vi "Main.vi"() -> ()   [LabVIEW 2014, in "CSV Analyzer.lvlib"]
uses:
  CSV Analyzer.lvlib
  <vilib>/SLL/SLL Table/SLL Table.lvclass
  <vilib>/Utility/error.llb/DialogType.ctl
  <vilib>/SLL/SLL Queued State Machine/Queue Driver/Create Queue.vi
  <vilib>/SLL/SLL Queued State Machine/Queue Driver/Enqueue an Item to Queue.vi
  <vilib>/SLL/SLL Queued State Machine/Queue Driver/Dequeue Queue.vi
  <vilib>/Utility/file.llb/Read From Spreadsheet File (string).vi
  <vilib>/SLL/SLL Queued State Machine/Queue Driver/Enqueue N Items.vi
  <vilib>/SLL/SLL Queued State Machine/Queue Driver/Flush Queue.vi
  <vilib>/SLL/SLL Queued State Machine/Queue Driver/Release Queue.vi
  <vilib>/SLL/SLL Queued State Machine/SLL QSM.lvlib
  <vilib>/SLL/SLL Spreadsheet/SLL Spreadsheet.lvlib
panel:
  in  "Delimiter":string(combo)=","
  in  "Use LabVIEW File Read?":bool
  in  "CSV File Path":path
  out "Total Columns":i32
  out "Total Rows":i32
  in  "Headers to List[]":string[](array[combo])
  in  "Filters":T1(array[cluster])
  out "Status":string
  in  "Analyze":bool
  out "Displayed Column Count":i32
  out "Displayed Row Count":i32
  in  "Mini Table":bool
  in  "2D Data Out[][]":i32(listbox)
  # "CSV Analyzer"
  # "Empty: Displays All Columns"
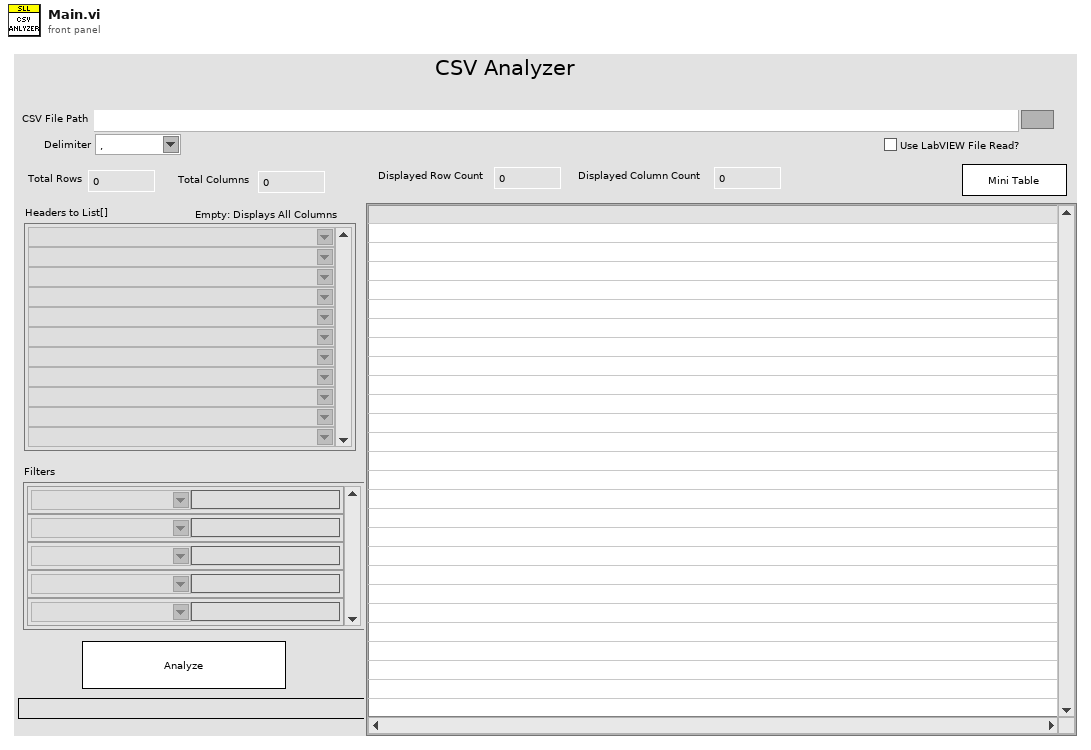
[diagram p1: front panel]
types:
  T1 = cluster{"Enable?":string, "Column Name":string}[]
  T2 = cluster{"Flags":cluster{"Source Code?":bool}, "SLL Table":refnum<class "SLL Table.lvclass">, "Headers[]":string[]}
  T3 = typedef "DialogType.ctl" = u16
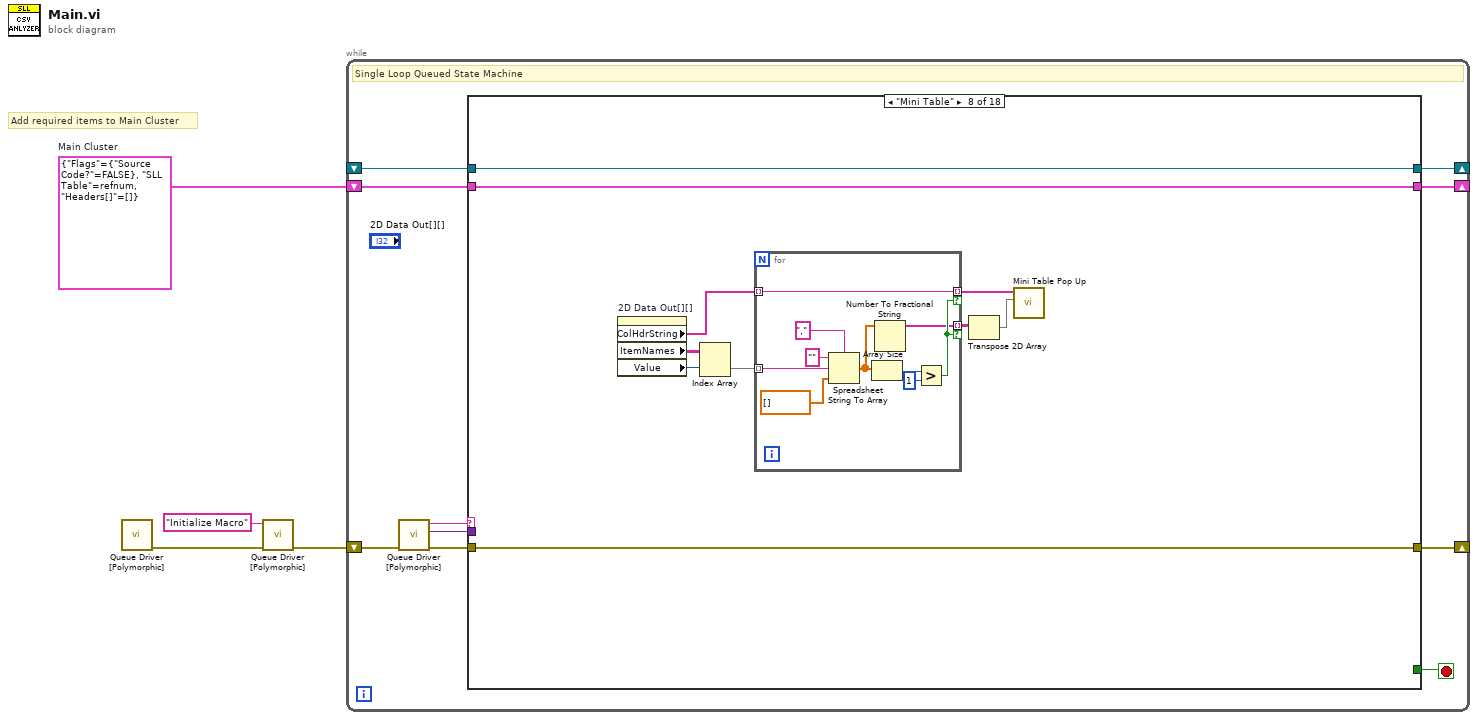
[diagram p0: block diagram]
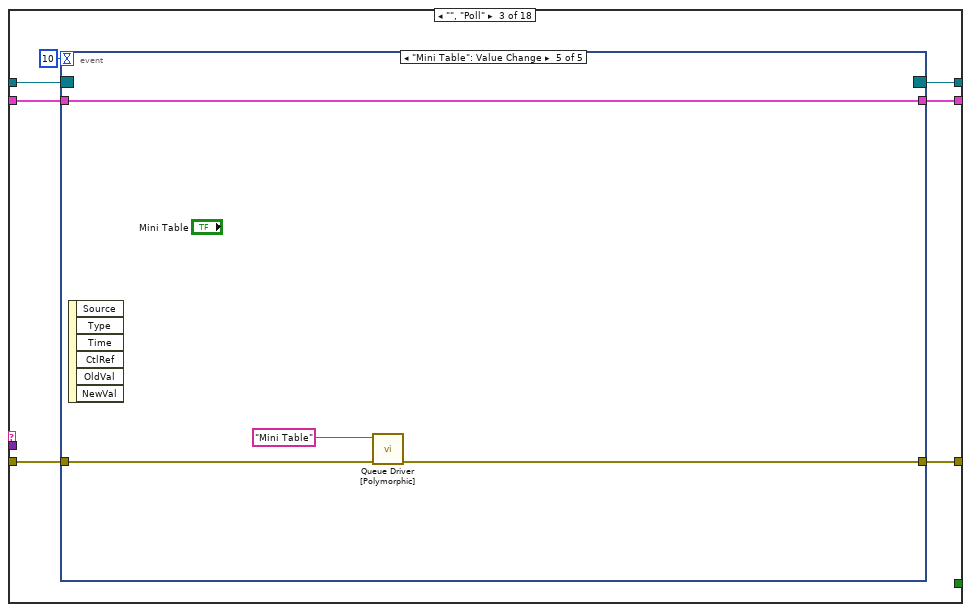
[diagram p4: hidden frame]
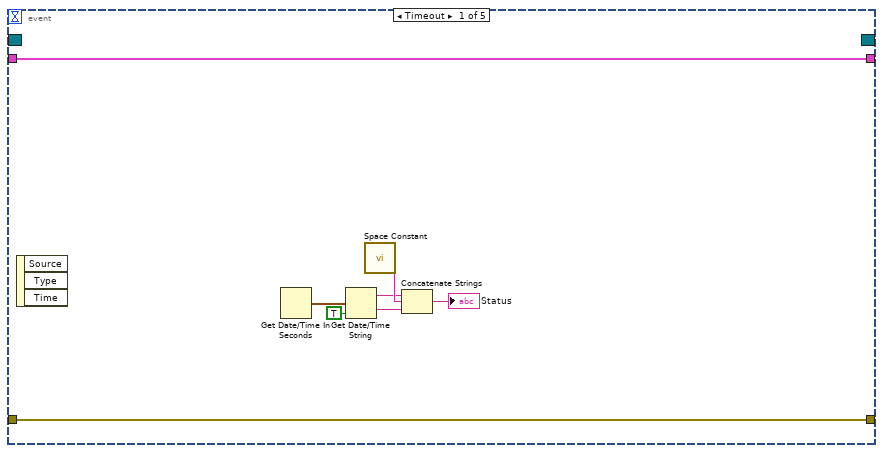
[diagram p5: hidden frame]
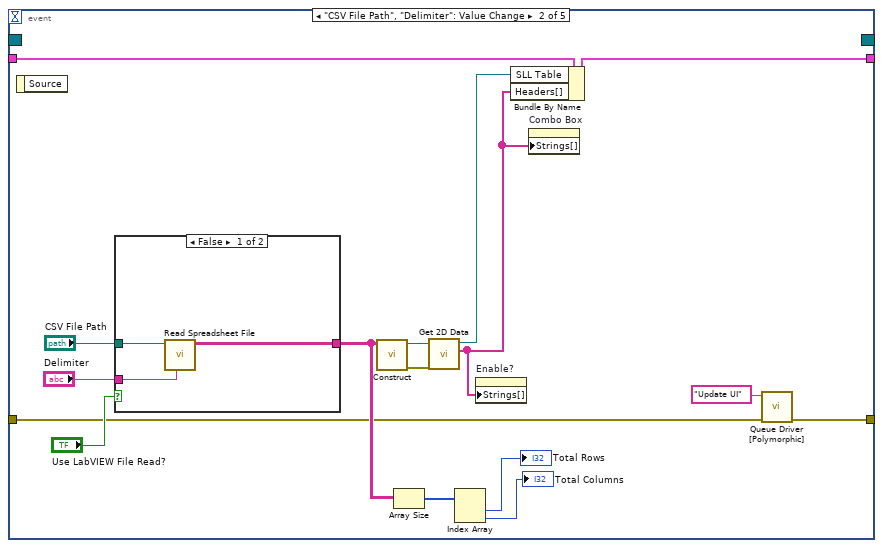
[diagram p6: hidden frame]
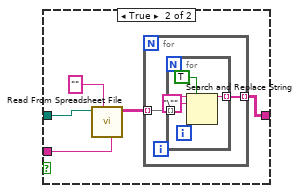
[diagram p7: hidden frame]
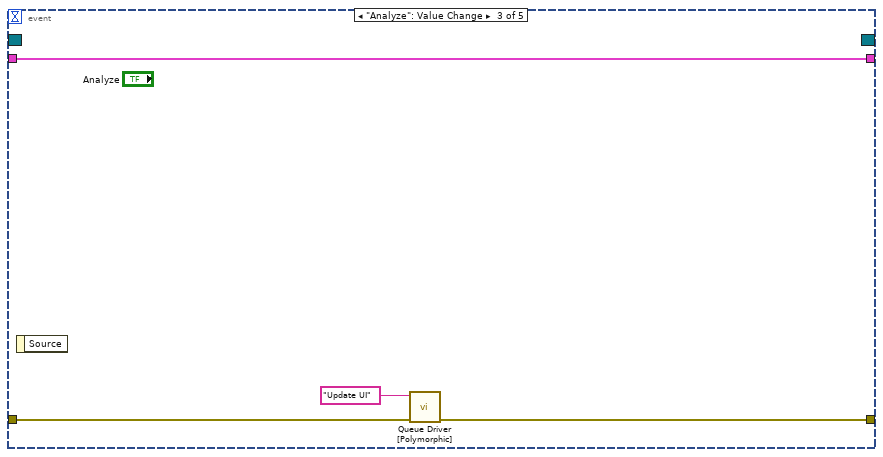
[diagram p8: hidden frame]
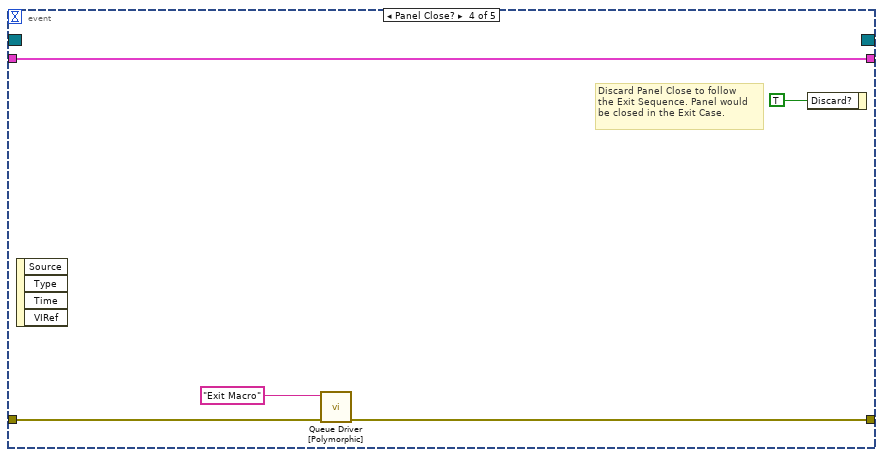
[diagram p9: hidden frame]
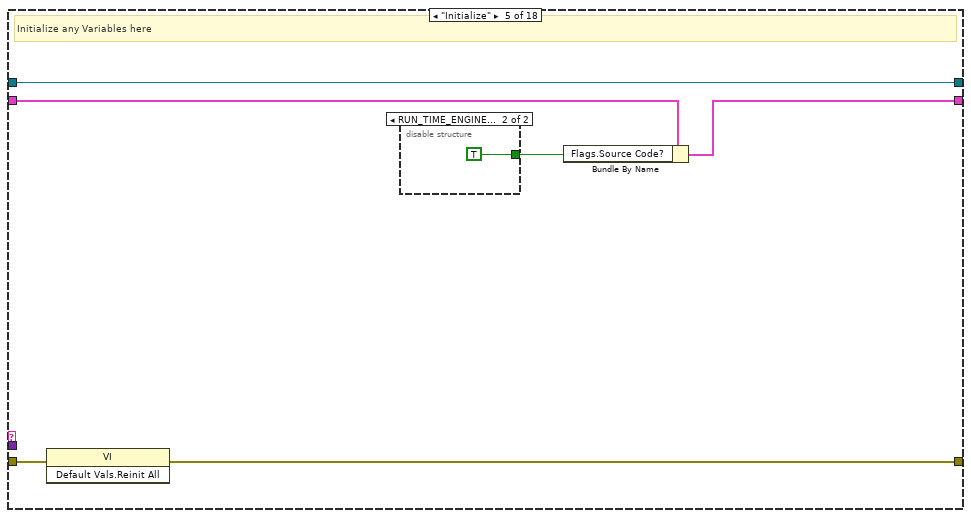
[diagram p11: hidden frame]
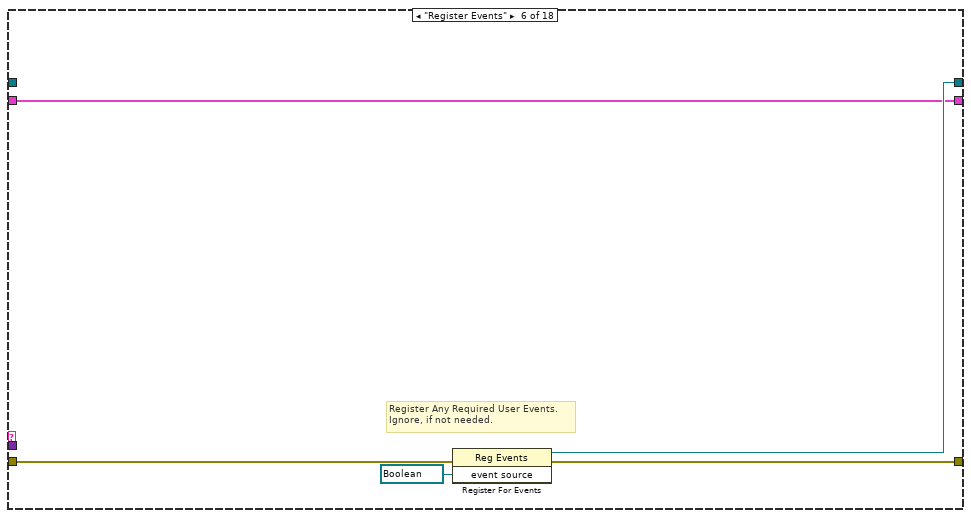
[diagram p13: hidden frame]
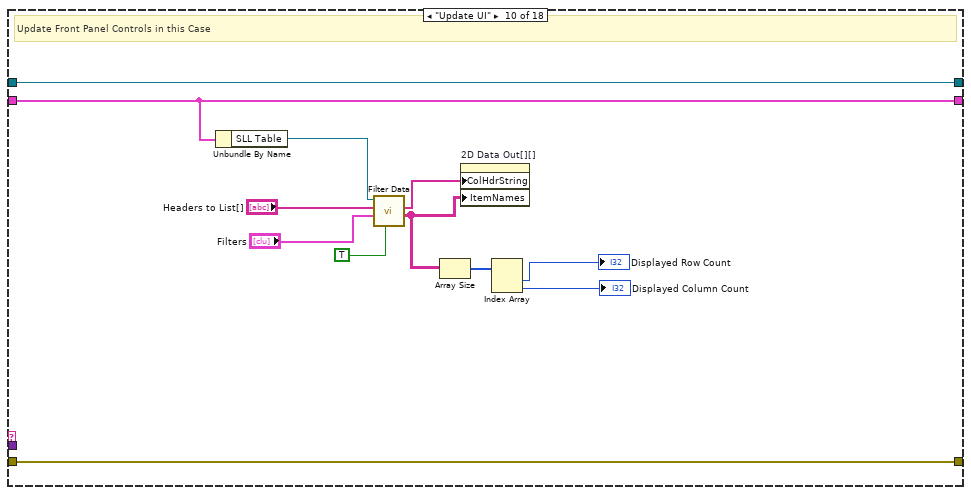
[diagram p16: hidden frame]
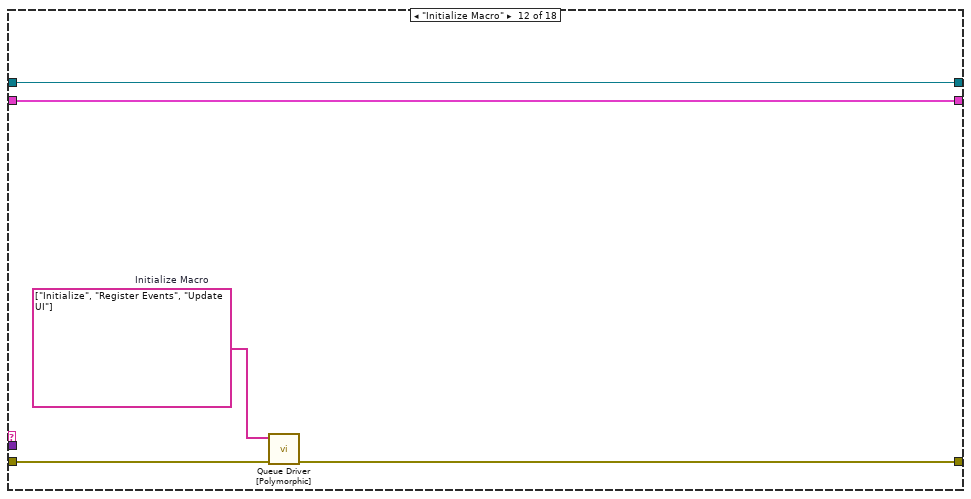
[diagram p18: hidden frame]
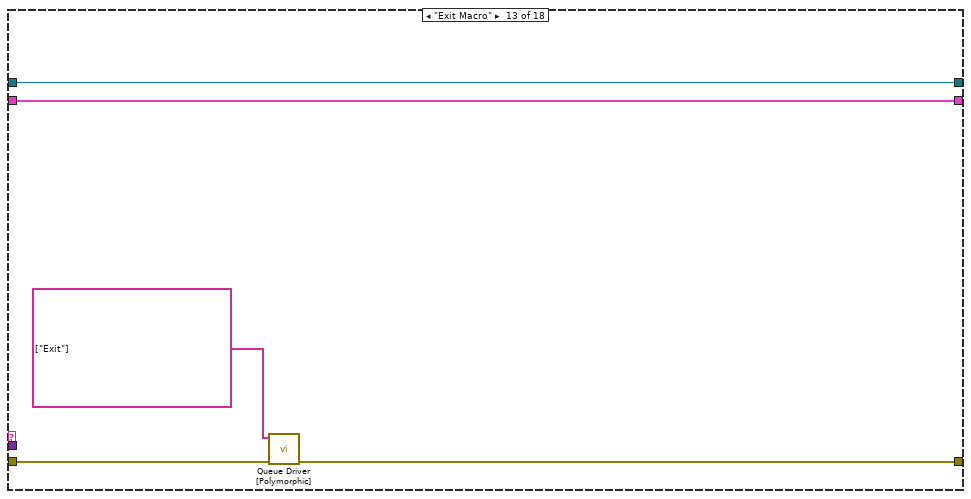
[diagram p19: hidden frame]
diagram:
  w3 = T2 {"Flags"={"Source Code?"=FALSE}, "SLL Table"=refnum, "Headers[]"=[]}  # Main Cluster
  # "Add required items to Main Cluster"
  n1 = call-poly <vilib>:"Queue Driver [Polymorphic].vi"() -> ("Error Out"=w2:errorcluster)  [unwired: 11 in]
  n2 = call-poly <vilib>:"Queue Driver [Polymorphic].vi"("Error In"=w2, "Item to Add"="Initialize Macro") -> ("Error Out"=w1:errorcluster)  [unwired: 9 in]
  n3 = while "SLL Queued State Machine" {
    shift-right: [w12] -> _
    shift-left: w1 -> [w14]
    shift-right: [w9] -> _
    shift-left: _ -> [w8]
    shift-right: [w7] -> _
    shift-left: w3 -> [w6]
    stop <- w11 stop-if-true
    # "Single Loop Queued State Machine"
    n4 = call-poly <vilib>:"Queue Driver [Polymorphic].vi"("Error In"=w14) -> ("Error Out"=w13:errorcluster, "Data"=w5:variant, "Dequeue"=w10:string)  [unwired: 8 in]
    n5 = case "QSM Case Structure" shown="\"Mini Table\"" w10 {
      selector: w10 -> [_ _ _ _ _ _ _ _ _ _ _ _ _ _ w151 _ _ _]
      tunnel: w13 -> [w17 w20 w25 w81 w82 w93 w96 w106 w119 w131 w134 w137 w142 w147 w150 w163 w166 w179]
      tunnel: [w17 w20 w26 w81 w83 w92 w96 w106 w119 w131 w134 w136 w141 w147 w154 w161 w166 w175] -> w12
      tunnel: [_ _ _ _ _ _ _ _ _ _ _ _ _ _ _ _ _ TRUE] -> w11
      tunnel: [w16 w19 w24 w80 w87 w91 w95 w105 w118 w130 w133 w139 w144 w146 w157 w160 w165 w178] -> w9
      tunnel: w8 -> [w16 w19 w23 w80 w87 _ w95 w105 w118 w130 w133 w139 w144 w146 w157 w160 w165 w178]
      tunnel: [w15 w18 w21 w79 w84 w90 w94 w104 w117 w120 w132 w138 w143 w145 w156 w159 w164 w177] -> w7
      tunnel: w6 -> [w15 w18 w22 w79 w85 w90 w94 w104 w117 w120 w132 w138 w143 w145 w156 w159 w164 w177]
      tunnel: w5 -> [_ _ _ _ _ _ _ _ _ _ _ _ _ _ _ _ _ _]
      frame "/--------------- Read Me -----------------/" {
        # "General Purpose Queue Based State Machine for Any Use Case (main application, module, pop up message etc)\n\nAdvantages:\n1. No Need to Pass Queue References between Queue Driver VIs.\n2. This template can be safely used in multiple parallel running modules without any issues.\n3. This template can also be safely used even in cases where the VI is configured to be a Clone, where multiple \ninstances of the VI could be executing concurrently.\n\nHow to Use:\n1. Add necessary items to the Main Cluster.\n2. Use the Polymorphic Queue Driver for doing any queue operations. There is no need to pass the queue driver\nreference, as the Queue Driver automatically infers the reference based on the VI instance from which it is called.\n3. Add any required user events in the \"Register Events\" case. Ignore if not needed.\n4. Use \"Sequences\" section for defining any list of state calls, which could be used in multiple places. \nEg: Initialize Sequence, might be needed if we need to any reinitialization."
      }
      frame "/------------------ Poll -------------------/" {
      }
      frame "", "Poll" {
        n6 = event shown="[4] \"Mini Table\": Value Change" {
          selector: w23 -> [_ _ _ _ _]
          dyn-events: [_ _ _ _ _] -> w24
          timeout: 10 -> [_ _ _ _ _]
          tunnel: [w35 w36 w67 w73 w77] -> w26
          tunnel: w25 -> [w35 w37 w66 w74 w78]
          tunnel: w22 -> [w34 w47 w69 w72 w76]
          tunnel: [w34 w49 w69 w72 w76] -> w21
          event Timeout {
            n7 = event-data() -> ()  [unwired: 1 in, 3 out]
            n8 = Get Date/Time In Seconds() -> (seconds since 1Jan1904=w33:timestamp)
            n9 = Get Date/Time String(seconds (now)=w33, want seconds? (F)=TRUE) -> (date string=w29:string, time string=w28:string)  [unwired: 1 in]
            n10 = call <vilib>:"Space Constant.vi"() -> ("String"=w30:string)
            n11 = Concatenate Strings(w29, w30, w28) -> (→"Status":string)
          }
          event "CSV File Path", "Delimiter": Value Change {
            n12 = event-data() -> ()  [unwired: 1 in, 1 out]
            n13 = case shown="False" "Use LabVIEW File Read?" {
              tunnel: [w54 w56] -> w45
              tunnel: "CSV File Path" -> [w53 w59]
              tunnel: "Delimiter" -> [w52 w55]
              frame False {
                n14 = call <vilib>:"Read Spreadsheet File.vi"("Delimiter (tab)"=w52, "File Path"=w53) -> ("2D Array"=w54:string[][])  [unwired: 8 in, 1 out]
              }
              frame True {
                n15 = call-poly <vilib>:"Read From Spreadsheet File.vi"("delimiter (\\t)"=w55, "format (%s)"="", "file path (dialog if empty)"=w59) -> ("all rows"=w57:string[][])  [unwired: 4 in, 4 out]
                n16 = for {
                  tunnel: w57 -> [w61] mode=indexing
                  tunnel: [w60] -> w56 mode=indexing
                  n17 = for {
                    tunnel: w61 -> [w65] mode=indexing
                    tunnel: [w63] -> w60 mode=indexing
                    n18 = Search and Replace String(replace all?=TRUE ("replace all? (F)"), input string=w65, search string="\"") -> (result string=w63:string)  [unwired: 5 in, 3 out]
                  }
                }
              }
            }
            n19 = call <vilib>:"Construct.vi"("2D String with Headers"=w45) -> ("error out"=w51:errorcluster, "SLL Spreadsheet"=w50:refnum<class "SLL Table.lvclass">)  [unwired: 9 in]
            n20 = Array Size(array=w45) -> (size(s)=w44:i32[])
            n21 = call <vilib>:"Get 2D Data.vi"("error in (no error)"=w51, "SLL Spreadsheet in"=w50) -> ("Headers Out[]"=w39:string[], "SLL Spreadsheet out"=w48:refnum<class "SLL Table.lvclass">)  [unwired: 6 in, 2 out]
            n22 = Index Array(array=w44) -> (element #1=→"Total Rows":i32, element #2=→"Total Columns":i32)  [unwired: 2 in]
            n23 = property on="Enable?" class="CmbBox"("Strings[]"=w39) -> ()  [unwired: 2 in, 2 out]
            n24 = Bundle By Name(cluster=w47, "SLL Table"=w48, "Headers[]"=w39) -> (w49:T2)
            n25 = property on="Combo Box" class="CmbBox"("Strings[]"=w39) -> ()  [unwired: 2 in, 2 out]
            n26 = call-poly <vilib>:"Queue Driver [Polymorphic].vi"("Error In"=w37, "Item to Add"="Update UI" ("Enqueue")) -> ("Error Out"=w36:errorcluster)  [unwired: 9 in]
          }
          event "Analyze": Value Change {
            n27 = event-data() -> ()  [unwired: 1 in, 1 out]
            n28 = call-poly <vilib>:"Queue Driver [Polymorphic].vi"("Error In"=w66, "Item to Add"="Update UI" ("Enqueue")) -> ("Error Out"=w67:errorcluster)  [unwired: 9 in]
          }
          event Panel Close? {
            # "Discard Panel Close to follow\nthe Exit Sequence. Panel would\nbe closed in the Exit Case."
            n29 = event-data() -> ()  [unwired: 1 in, 4 out]
            n30 = call-poly <vilib>:"Queue Driver [Polymorphic].vi"("Error In"=w74, "Item to Add"="Exit Macro" ("Enqueue")) -> ("Error Out"=w73:errorcluster)  [unwired: 9 in]
            n31 = event-data("Discard?"=TRUE) -> ()  [unwired: 1 in, 1 out]
          }
          event "Mini Table": Value Change {
            n32 = event-data() -> ()  [unwired: 1 in, 6 out]
            n33 = call-poly <vilib>:"Queue Driver [Polymorphic].vi"("Error In"=w78, "Item to Add"="Mini Table" ("Enqueue")) -> ("Error Out"=w77:errorcluster)  [unwired: 9 in]
          }
        }
      }
      frame "/--------------- Initialize -----------------/" {
      }
      frame "Initialize" {
        # "Initialize any Variables here"
        n34 = invoke class="VI" method="Default Vals.Reinit All"(error in=w82) -> (error out=w83:errorcluster)  [unwired: 2 in, 2 out]
        n35 = disable-structure shown="RUN_TIME_ENGINE==False" {
          disable-tunnel: [_ TRUE] -> w86
          frame condition #0 {
          }
          frame condition #1 (active) {
          }
        }
        n36 = Bundle By Name(cluster=w85, "Flags.Source Code?"=w86) -> (w84:T2)
      }
      frame "Register Events" {
        # "Register Any Required User Events. \nIgnore, if not needed."
        n37 = register-events(error in=w93, refnum<vi> refnum ("event source")) -> (reference out=w91:refnum<event-registration>, error out=w92:errorcluster)  [unwired: 1 in]
      }
      frame "/---------- Custom Case Splitter ----------/" {
      }
      frame "Mini Table" {
        n38 = property on="2D Data Out[][]" class="MCListbox (strict)"() -> ("ColHdrString"=w100:string[], "ItemNames"=w103:string[][], "Value"=w102:i32)  [unwired: 2 in, 2 out]
        n39 = Index Array(array=w103, index (row)=w102) -> (element=w101:string[])  [unwired: 1 in]
        n40 = for {
          tunnel: w101 -> [w116] mode=indexing
          tunnel: w100 -> [w110] mode=indexing
          tunnel: [w107] -> w98 mode=indexing if=w109
          tunnel: [w110] -> w99 mode=indexing if=w109
          n41 = Spreadsheet String To Array(delimiter (Tab)=",", format string="", spreadsheet string=w116, array type (2D Dbl)=dbl[] []) -> (array=w111:dbl[])
          n42 = Array Size(array=w111) -> (size(s)=w113:i32)
          n43 = Number To Fractional String(number=w111) -> (F-format string=w107:string[])  [unwired: 3 in]
          n44 = Greater?(x=w113, y=1) -> (0:w109:bool)
        }
        n45 = Transpose 2D Array(2D array=w98) -> (transposed array=w97:string[][])
        n46 = call "Mini Table Pop Up.vi"("Data[][]"=w97, "Headers[]"=w99) -> ()  [unwired: 9 in, 1 out]
      }
      frame "/-------------- User Interface --------------/" {
        # "Duplicate this case to create additional case splitters for readability"
      }
      frame "Update UI" {
        # "Update Front Panel Controls in this Case"
        n47 = Unbundle By Name(w120) -> ("SLL Table"=w129:refnum<class "SLL Table.lvclass">)
        n48 = call <vilib>:"Filter Data.vi"("Count? (F)"=TRUE, "Value Filters[]"="Filters", "Header Order[]"="Headers to List[]", "SLL Table in"=w129) -> ("2D Data Out[][]"=w121:string[][], "Headers Out[]"=w127:string[])  [unwired: 4 in, 2 out]
        n49 = Array Size(array=w121) -> (size(s)=w126:i32[])
        n50 = property on="2D Data Out[][]" class="MCListbox (strict)"("ColHdrString"=w127, "ItemNames"=w121) -> ()  [unwired: 2 in, 2 out]
        n51 = Index Array(array=w126) -> (element #1=→"Displayed Row Count":i32, element #2=→"Displayed Column Count":i32)  [unwired: 2 in]
      }
      frame "/----------------- Macros -----------------/" {
      }
      frame "Initialize Macro" {
        w135 = string[] ["Initialize", "Register Events", "Update UI"]  # Initialize Macro
        n52 = call-poly <vilib>:"Queue Driver [Polymorphic].vi"("Error In"=w137, "Enqueue N"=w135) -> ("Error Out"=w136:errorcluster)  [unwired: 9 in]
      }
      frame "Exit Macro" {
        n53 = call-poly <vilib>:"Queue Driver [Polymorphic].vi"("Error In"=w142, "Enqueue N"=string[] ["Exit"]) -> ("Error Out"=w141:errorcluster)  [unwired: 9 in]
      }
      frame "/-------------- Error Handler--------------/" {
      }
      frame Default {
        # "Undefined Case/Spelling Errors - Show Message to Developer"
        n54 = property class="VI"(error in=w150) -> (error out=w149:errorcluster, "Name"=w148:string)  [unwired: 1 in, 1 out]
        n55 = Format Into String(format string="\"%s\" in the VI - %s" ("message"), initial string="Undefined case - ", error in=w149, w151, w148) -> (resulting string=w152:string, error out=w154:errorcluster)
        n56 = One Button Dialog(message=w152) -> ()  [unwired: 1 in, 1 out]
      }
      frame "Error" {
        w158 = T3 2 items=["no dialog", "OK message", "continue or stop message", "OK message + warnings", "continue/stop + warnings"] ("type of dialog (OK msg:1)")
        # "Handle the Error"
        n57 = call <vilib>:"Simple Error Handler.vi"("type of dialog (OK msg:1)"=w158, "error in (no error)"=w163) -> ("error out"=w162:errorcluster)  [unwired: 3 in, 4 out]
        n58 = call <vilib>:"Clear Errors.vi"("error in (no error)"=w162) -> ("error out"=w161:errorcluster)  [unwired: 5 in, 1 out]
      }
      frame "/------------------- Exit --------------------/" {
      }
      frame "Exit" {
        n59 = call-poly <vilib>:"Queue Driver [Polymorphic].vi"("Error In"=w179) -> ("Error Out"=w180:errorcluster)  [unwired: 9 in, 1 out]
        n60 = Unbundle By Name(w177) -> ("Flags.Source Code?"=w170:bool)
        n61 = call-poly <vilib>:"Queue Driver [Polymorphic].vi"("Error In"=w180) -> ("Error Out"=w176:errorcluster)  [unwired: 10 in]
        n62 = Call Chain() -> (call chain=w174:string[])
        n63 = Array Size(array=w174) -> (size(s)=w173:i32)
        n64 = Equal?(x=w173, y=1) -> (x = y?=w171:bool)
        n65 = And(x=w170, y=w171) -> (x .and. y?=w169:bool)
        n66 = case "Skip Panel Close when in Source\nCode and is the top most caller" shown="True" w169 {
          tunnel: w176 -> [w183 w185]
          tunnel: [w184 w185] -> w175
          frame False {
            # "Close Panel"
            n67 = invoke class="VI" method="FP.Close"() -> (error out=w182:errorcluster)  [unwired: 3 in, 2 out]
            n68 = Merge Errors(w183, w182) -> (w184:errorcluster)
          }
          frame True {
            # "Do Not Close Panel"
          }
        }
        n69 = property on="2D Data Out[][]" class="MCListbox (strict)"("ColHdrString"=string[] [] ("Column Header Strings[]"), "ItemNames"=string[][] [] ("2D Data Out[][] 2")) -> ()  [unwired: 2 in, 2 out]
      }
    }
  }
